vi "map js test.vi"() -> ()   [LabVIEW 2015]
panel:
  in  "stop":bool
  in  "Clear markers":bool
  in  "WebBrowser":refnum<k7>(container)
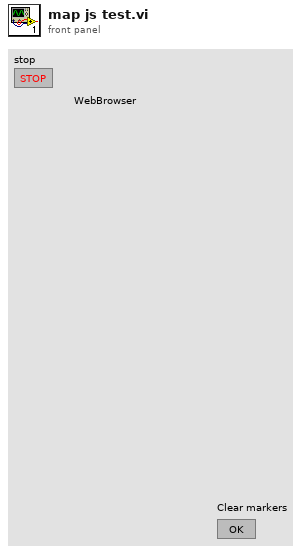
[diagram p1: front panel]
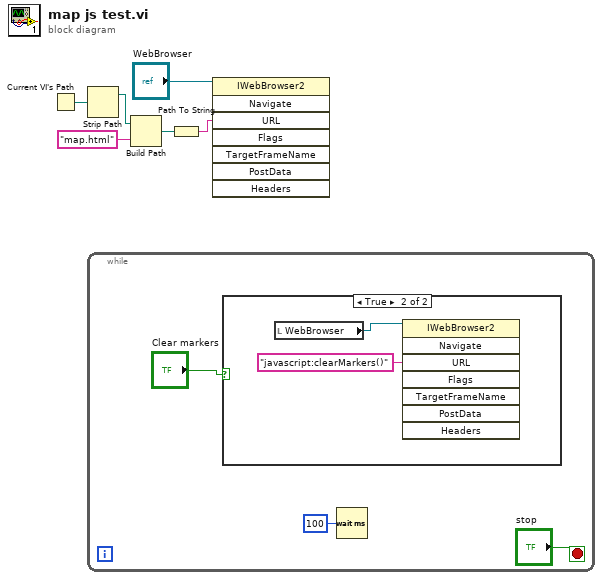
[diagram p0: block diagram]
diagram:
  n1 = Current VI's Path() -> (path=w6:path)
  n2 = Strip Path(path=w6) -> (stripped path=w5:path)  [unwired: 1 out]
  n3 = while {
    stop <- "stop" stop-if-true
    n4 = case shown="True" "Clear markers" {
      frame False {
      }
      frame True {
        n5 = local read "WebBrowser"() -> (w10:refnum<k7>)
        n6 = invoke class="IWebBrowser2" method="Navigate"(reference=w10, "URL"="javascript:clearMarkers()") -> ()  [unwired: 6 in, 8 out]
      }
    }
    n7 = Wait (ms)(milliseconds to wait=u32 100) -> ()  [unwired: 1 out]
  }
  n8 = Build Path(base path=w5, name or relative path="map.html") -> (appended path=w2:path)
  n9 = Path To String(path=w2) -> (string=w1:string)
  n10 = invoke class="IWebBrowser2" method="Navigate"(reference="WebBrowser", "URL"=w1) -> ()  [unwired: 6 in, 8 out]
